vi "AssertsLess.vi"(11 "error in (no error)":errorcluster) -> (15 "error out":errorcluster)   [LabVIEW 2016, in "DronaTest.lvlib"]
uses:
  APIs/Assert/AssertControlValue/LessOrEqual.vi
  <vilib>/addons/_JKI Toolkits/Caraya/classes/Assert/Assert Not Error.vi
  APIs/Assert/AssertControlValue/Less.vi
  <vilib>/addons/_JKI Toolkits/Caraya/classes/Assert/Assert Error.vi
  DronaTest.lvlib
  <vilib>/addons/_JKI Toolkits/Caraya/classes/Test/Test.lvclass
  Drona.lvlib
  <vilib>/addons/_JKI Toolkits/Caraya/classes/Assert/Assert.lvclass
  APIs/Assert/AssertControlValue/AssertControlValue.lvlib
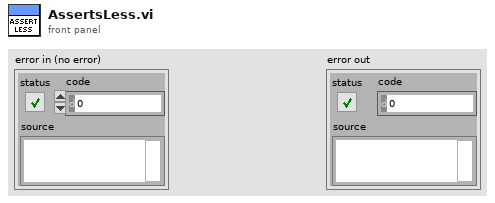
[diagram p1: front panel]
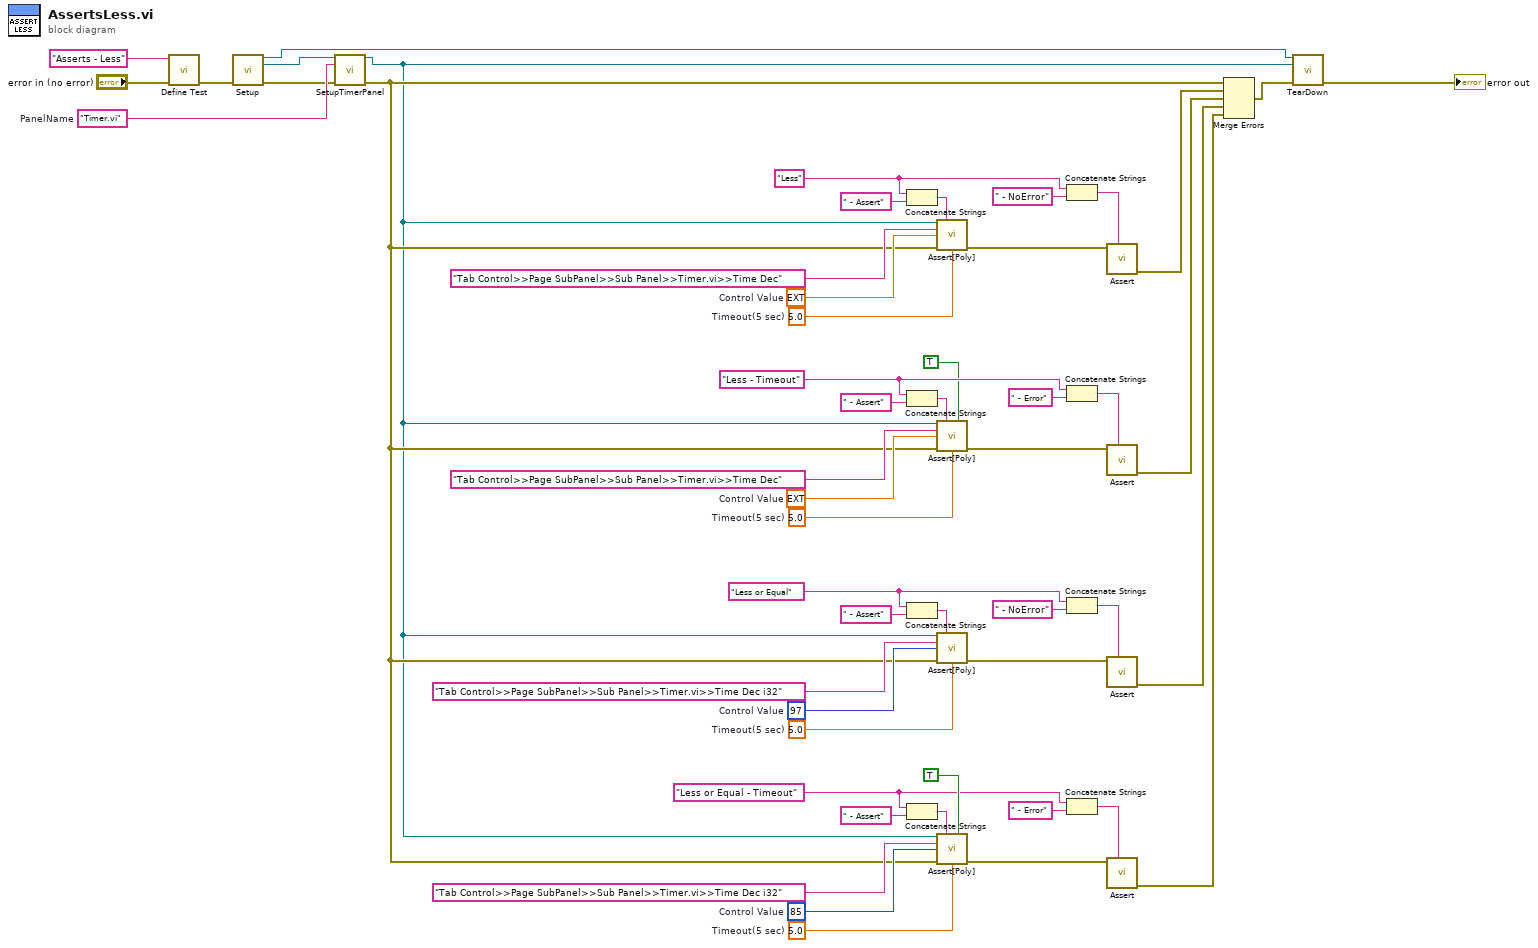
[diagram p0: block diagram]
diagram:
  w9 = "Timer.vi"  # PanelName
  w41 = 5.0  # Timeout(5 sec)
  w40 = 97  # Control Value
  w39 = "Less or Equal" ("string")
  w42 = 5.0  # Timeout(5 sec)
  w43 = 85  # Control Value
  w44 = "Less or Equal - Timeout" ("string")
  w24 = 5.0  # Timeout(5 sec)
  w25 = ext 97.0  # Control Value
  w26 = "Less" ("string")
  w23 = 5.0  # Timeout(5 sec)
  w22 = ext 85.0  # Control Value
  w21 = "Less - Timeout" ("string")
  n1 = call <vilib>:"Define Test.vi"("error in (no error)"="error in (no error)", "Label (VI Title)"="Asserts - Less") -> ("error out"=w4:errorcluster)  [unwired: 9 in]
  n2 = call "Setup.vi"("error in (no error)"=w4) -> ("Application Ref"=w3:refnum<vi>, "VI out"=w7:refnum<vi>, "error out"=w8:errorcluster)  [unwired: 12 in]
  n3 = call "SetupTimerPanel.vi"("VI in"=w7, "Panel Name"=w9, "error in (no error)"=w8) -> ("VI out"=w1:refnum<vi>, "error out"=w2:errorcluster)  [unwired: 11 in]
  n4 = Concatenate Strings(w26, " - Assert" ("string")) -> (w28:string)
  n5 = Concatenate Strings(w21, " - Assert" ("string")) -> (w19:string)
  n6 = Concatenate Strings(w39, " - Assert" ("string")) -> (w37:string)
  n7 = Concatenate Strings(w44, " - Assert" ("string")) -> (w46:string)
  n8 = call-poly "Assert[Poly].vi"("VI Reference In"=w1, "Test Label"=w28, "Control Path"="Tab Control>>Page SubPanel>>Sub Panel>>Timer.vi>>Time Dec", "Control Value"=w25, "Error In"=w2, "Timeout(5 sec)"=w24) -> ("Error Out"=w29:errorcluster)  [unwired: 8 in, 1 out]
  n9 = call-poly "Assert[Poly].vi"("VI Reference In"=w1, "Test Label"=w19, "Assert Only? (F)"=TRUE, "Control Path"="Tab Control>>Page SubPanel>>Sub Panel>>Timer.vi>>Time Dec", "Control Value"=w22, "Error In"=w2, "Timeout(5 sec)"=w23) -> ("Error Out"=w18:errorcluster)  [unwired: 7 in, 1 out]
  n10 = call-poly "Assert[Poly].vi"("VI Reference In"=w1, "Test Label"=w37, "Control Path"="Tab Control>>Page SubPanel>>Sub Panel>>Timer.vi>>Time Dec i32", "Control Value"=w40, "Error In"=w2, "Timeout(5 sec)"=w41) -> ("Error Out"=w36:errorcluster)  [unwired: 8 in, 1 out]
  n11 = call-poly "Assert[Poly].vi"("VI Reference In"=w1, "Test Label"=w46, "Assert Only? (F)"=TRUE, "Control Path"="Tab Control>>Page SubPanel>>Sub Panel>>Timer.vi>>Time Dec i32", "Control Value"=w43, "Error In"=w2, "Timeout(5 sec)"=w42) -> ("Error Out"=w47:errorcluster)  [unwired: 7 in, 1 out]
  n12 = Concatenate Strings(w26, " - NoError" ("string")) -> (w27:string)
  n13 = Concatenate Strings(w21, " - Error" ("string")) -> (w20:string)
  n14 = Concatenate Strings(w39, " - NoError" ("string")) -> (w38:string)
  n15 = Concatenate Strings(w44, " - Error" ("string")) -> (w45:string)
  n16 = call-poly <vilib>:"Assert.vi"("Label"=w27, "Not Error?"=w29) -> ("error out"=w13:errorcluster)  [unwired: 9 in]
  n17 = call-poly <vilib>:"Assert.vi"("Label"=w20, "Error?"=w18) -> ("error out"=w12:errorcluster)  [unwired: 9 in]
  n18 = call-poly <vilib>:"Assert.vi"("Label"=w38, "Not Error?"=w36) -> ("error out"=w11:errorcluster)  [unwired: 9 in]
  n19 = call-poly <vilib>:"Assert.vi"("Label"=w45, "Error?"=w47) -> ("error out"=w10:errorcluster)  [unwired: 9 in]
  n20 = Merge Errors(w2, w13, w12, w11, w10) -> (w6:errorcluster)
  n21 = call "TearDown.vi"("Application Ref"=w3, "VI in"=w1, "error in (no error)"=w6) -> ("error out"=→"error out":errorcluster)  [unwired: 12 in]
